vi "Begin.vi"(8 "error in":errorcluster) -> (0 "error out":errorcluster)   [LabVIEW 2019]
doc: "Called before other user functions, this VI is expected to open initial I/O refnums, load in file data, and do all program initialization. Notice that the <B>error out</B> terminal is simply used for data flow. Wiring it to other structures or subVIs ensures that this VI runs first."
uses:
  <vilib>/Rock Robotics/SystemInterfaces/DIO/FPGA_DIOPWMChannel.ctl
  Robot Global Data.vi
  <vilib>/Rock Robotics/WPI/DriverStation/WPI_DriverStationRobotMode2.ctl
  <vilib>/Rock Robotics/WPI/Joystick/WPI_JoystickDeviceEnum.ctl
  <vilib>/Rock Robotics/Network Tables/NT Write String Array.vi
  <vilib>/Rock Robotics/SystemInterfaces/AI/FPGA_AIGyroChannel.ctl
  <vilib>/Rock Robotics/SystemInterfaces/DIO/FPGA_DIOChannel.ctl
  <vilib>/Rock Robotics/WPI/Gyro/WPI_GyroAnalogOpen.vi
  <vilib>/Rock Robotics/WPI/ThirdParty/JAS_Junk/TrajLib/Trajectory_Library.lvlib
panel:
  in  "Tab Control":T1(tab)
  # "Instructions:\nThis should create a path, show the data on the various tabs and optionally write the motor demands and expected results to a file for use on a a robot..\n1) Enter robot data on Robot Data Tab\n2) Define your path definitions.\n3) Define the time increment.  0.020 is chosen since that matches the normal loop time.\n4) Press calculate path.  If a good path was calculated it will be displayed on the Tank Data tab, and the Ready to Execute will indicate execution can begin.\nThe path can be recalculated many times before selecting execute.\n\nTo write to a file.\n5) Select the file name\n6) This example uses \"steps\", sequential numbers for inclusion into a list based autonomous routine.  Including the step number if optional.\n7) This uses command numbers to indicate first, last, and intermediate steps.  This allows some simplification of the execution routine.  It\nalso allows the path to be executed backwards if desired.  The command numbers are changeable.\n8) Press \"Create Command List\".\n\nNotes:\n- PC robot simulataion is disabled in this program.  The code is still there if you want to restore it and try it out.  Use one of the other test programs \nto simulate the path on a PC.\n- The path generation logic doesn't account distribution of speed to the left and right wheels.  As a result the maximum speed can be exceeded.\nIf this happens, but Path Speed > Max light will light and Ready to Execute will not light.  Lower the maximum speed in the Robot Data tab\nand recalulate the path.\n- 2019 playing field size - width: 26 ft 11.25 In = 323.25 in , length: 52 ft 5.25 in = 629.25 in  (I didn't verify this for the 2020 version.)"
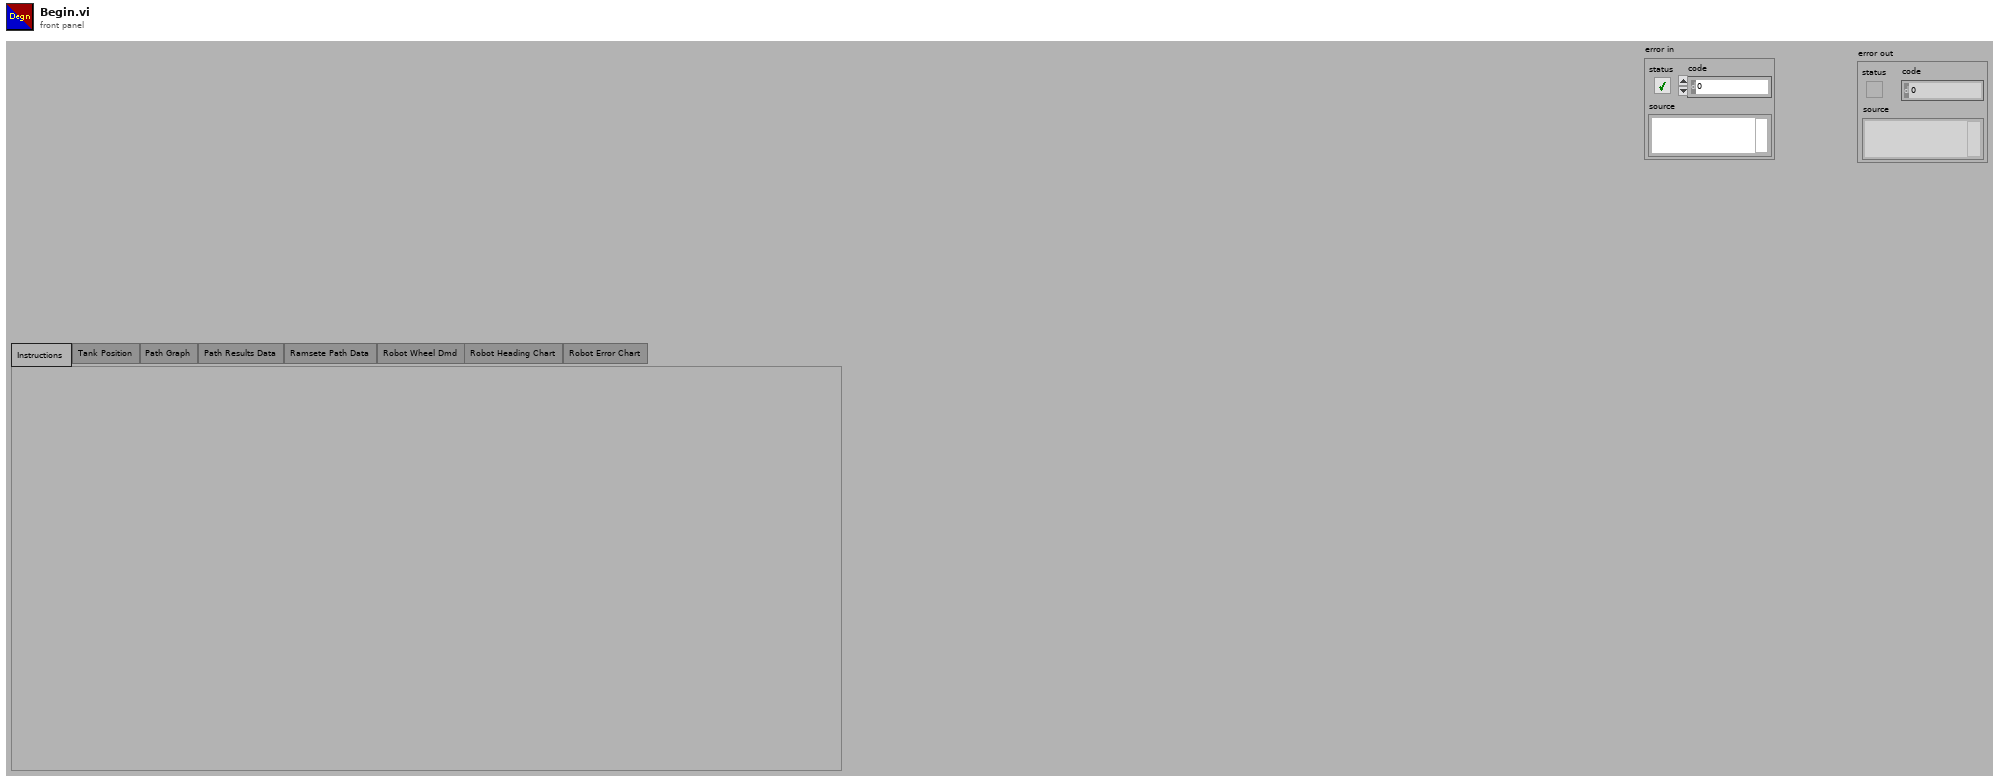
[diagram p1: front panel]
types:
  T1 = enum32{"Instructions", "Tank Position", "Path Graph", "Path Results Data", "Ramsete Path Data", "Robot Wheel Dmd", "Robot Heading Chart", "Robot Error Chart"}
  T2 = typedef "FPGA_DIOChannel.ctl" = enum8{"DIO 0", "DIO 1", "DIO 2", "DIO 3", "DIO 4", "DIO 5", "DIO 6", "DIO 7", "DIO 8", "DIO 9", "DIO MXP 0", "DIO MXP 1", "DIO MXP 2", "DIO MXP 3", "DIO MXP 4", "DIO MXP 5", "DIO MXP 6", "DIO MXP 7", "DIO MXP 8", "DIO MXP 9", "DIO MXP 10", "DIO MXP 11", "DIO MXP 12", "DIO MXP 13", "DIO MXP 14", "DIO MXP 15", "SPI Port CS1", "SPI Port CS2", "SPI Port CS3", "SPI Port MISO", "SPI Port MOSI", "Invalid"}
  T3 = typedef "FPGA_DIOPWMChannel.ctl" = enum8{"PWM 0", "PWM 1", "PWM 2", "PWM 3", "PWM 4", "PWM 5", "PWM 6", "PWM 7", "PWM 8", "PWM 9", "PWM MXP 0", "PWM MXP 1", "PWM MXP 2", "PWM MXP 3", "PWM MXP 4", "PWM MXP 5", "PWM MXP 6", "PWM MXP 7", "PWM MXP 8", "PWM MXP 9", "Invalid"}
  T4 = typedef "FPGA_AIGyroChannel.ctl" = enum8{"AI 0", "AI 1", "Invalid"}
  T5 = typedef "WPI_JoystickDeviceEnum.ctl" = enum16{"USB 0", "USB 1", "USB 2", "USB 3", "USB 4", "USB 5"}
  T6 = typedef "WPI_DriverStationRobotMode2.ctl" = enum16{"Autonomous Disabled", "Autonomous Enabled", "Teleop Disabled", "Teleop Enabled", "Disconnected", "Finish", "Test Disabled", "Test Enabled", "Emergency Stopped"}
  T7 = typedef "Trajectory_Library.lvlib/ROTATION2D.ctl" = cluster{"VALUE":dbl, "COS":dbl, "SIN":dbl}
  T8 = typedef "Trajectory_Library.lvlib/SWERVE_DRIVE_MODULE_POSITION.ctl" = cluster{"Distance":dbl, "Angle":T7, "P":bool}
  T9 = typedef "WPI_JoystickDevRef.ctl" = cluster{"Device":T5}
  T10 = typedef "WPI_GyroDevRef.ctl" = cluster{"DevStatus":errorcluster, "Analog Channel":T11, "Gain (VoltsPerDegree/Second)":dbl, "Gyro Type":enum16{"Analog", "XRS450"}, "Handle":i32, "SPI Bus":T12, "Device Found":bool, "Sample Rate":dbl, "Calibrate On Open":bool, "Offset":dbl}
  T11 = typedef "FPGA_AIChannel.ctl" = enum8{"AI 0", "AI 1", "AI 2", "AI 3", "AI MXP 0", "AI MXP 1", "AI MXP 2", "AI MXP 3", "Invalid"}
  T12 = typedef "spi_bus.ctl" = enum16{"SPI On-Board, CS0", "SPI On-Board, CS1", "SPI On-Board, CS2", "SPI On-Board, CS3", "SPI MXP", "Invalid"}
  T13 = typedef "Trajectory_Library.lvlib/TRANSLATION2D.ctl" = cluster{"X":dbl, "Y":dbl}
  T14 = typedef "Trajectory_Library.lvlib/POSE2D.ctl" = cluster{"TRANSLATION":T13, "ROTATION":T7}
  T15 = typedef "Trajectory_Library.lvlib/SWERVE_DRIVE_ODOMETRY.ctl" = cluster{"POSE":T14, "GyroOffset":T7, "PreviousAngle":T7, "PrevModulePositions":T8[], "NumModules":i32}
  T16 = typedef "Trajectory_Library.lvlib/SWERVE_DRIVE_KINEMATICS.ctl" = cluster{"NumModules":i32, "InverseKinematics":T17, "ForwardKinematics":T17, "Modules":T13[], "PrevCoR":T13, "SavedModuleStates":T18[]}
  T17 = typedef "NI_Matrix.lvlib/RealMatrix.ctl" = dbl[][]
  T18 = typedef "Trajectory_Library.lvlib/SWERVE_DRIVE_MODULE_STATE.ctl" = cluster{"Speed":dbl, "Angle":T7}
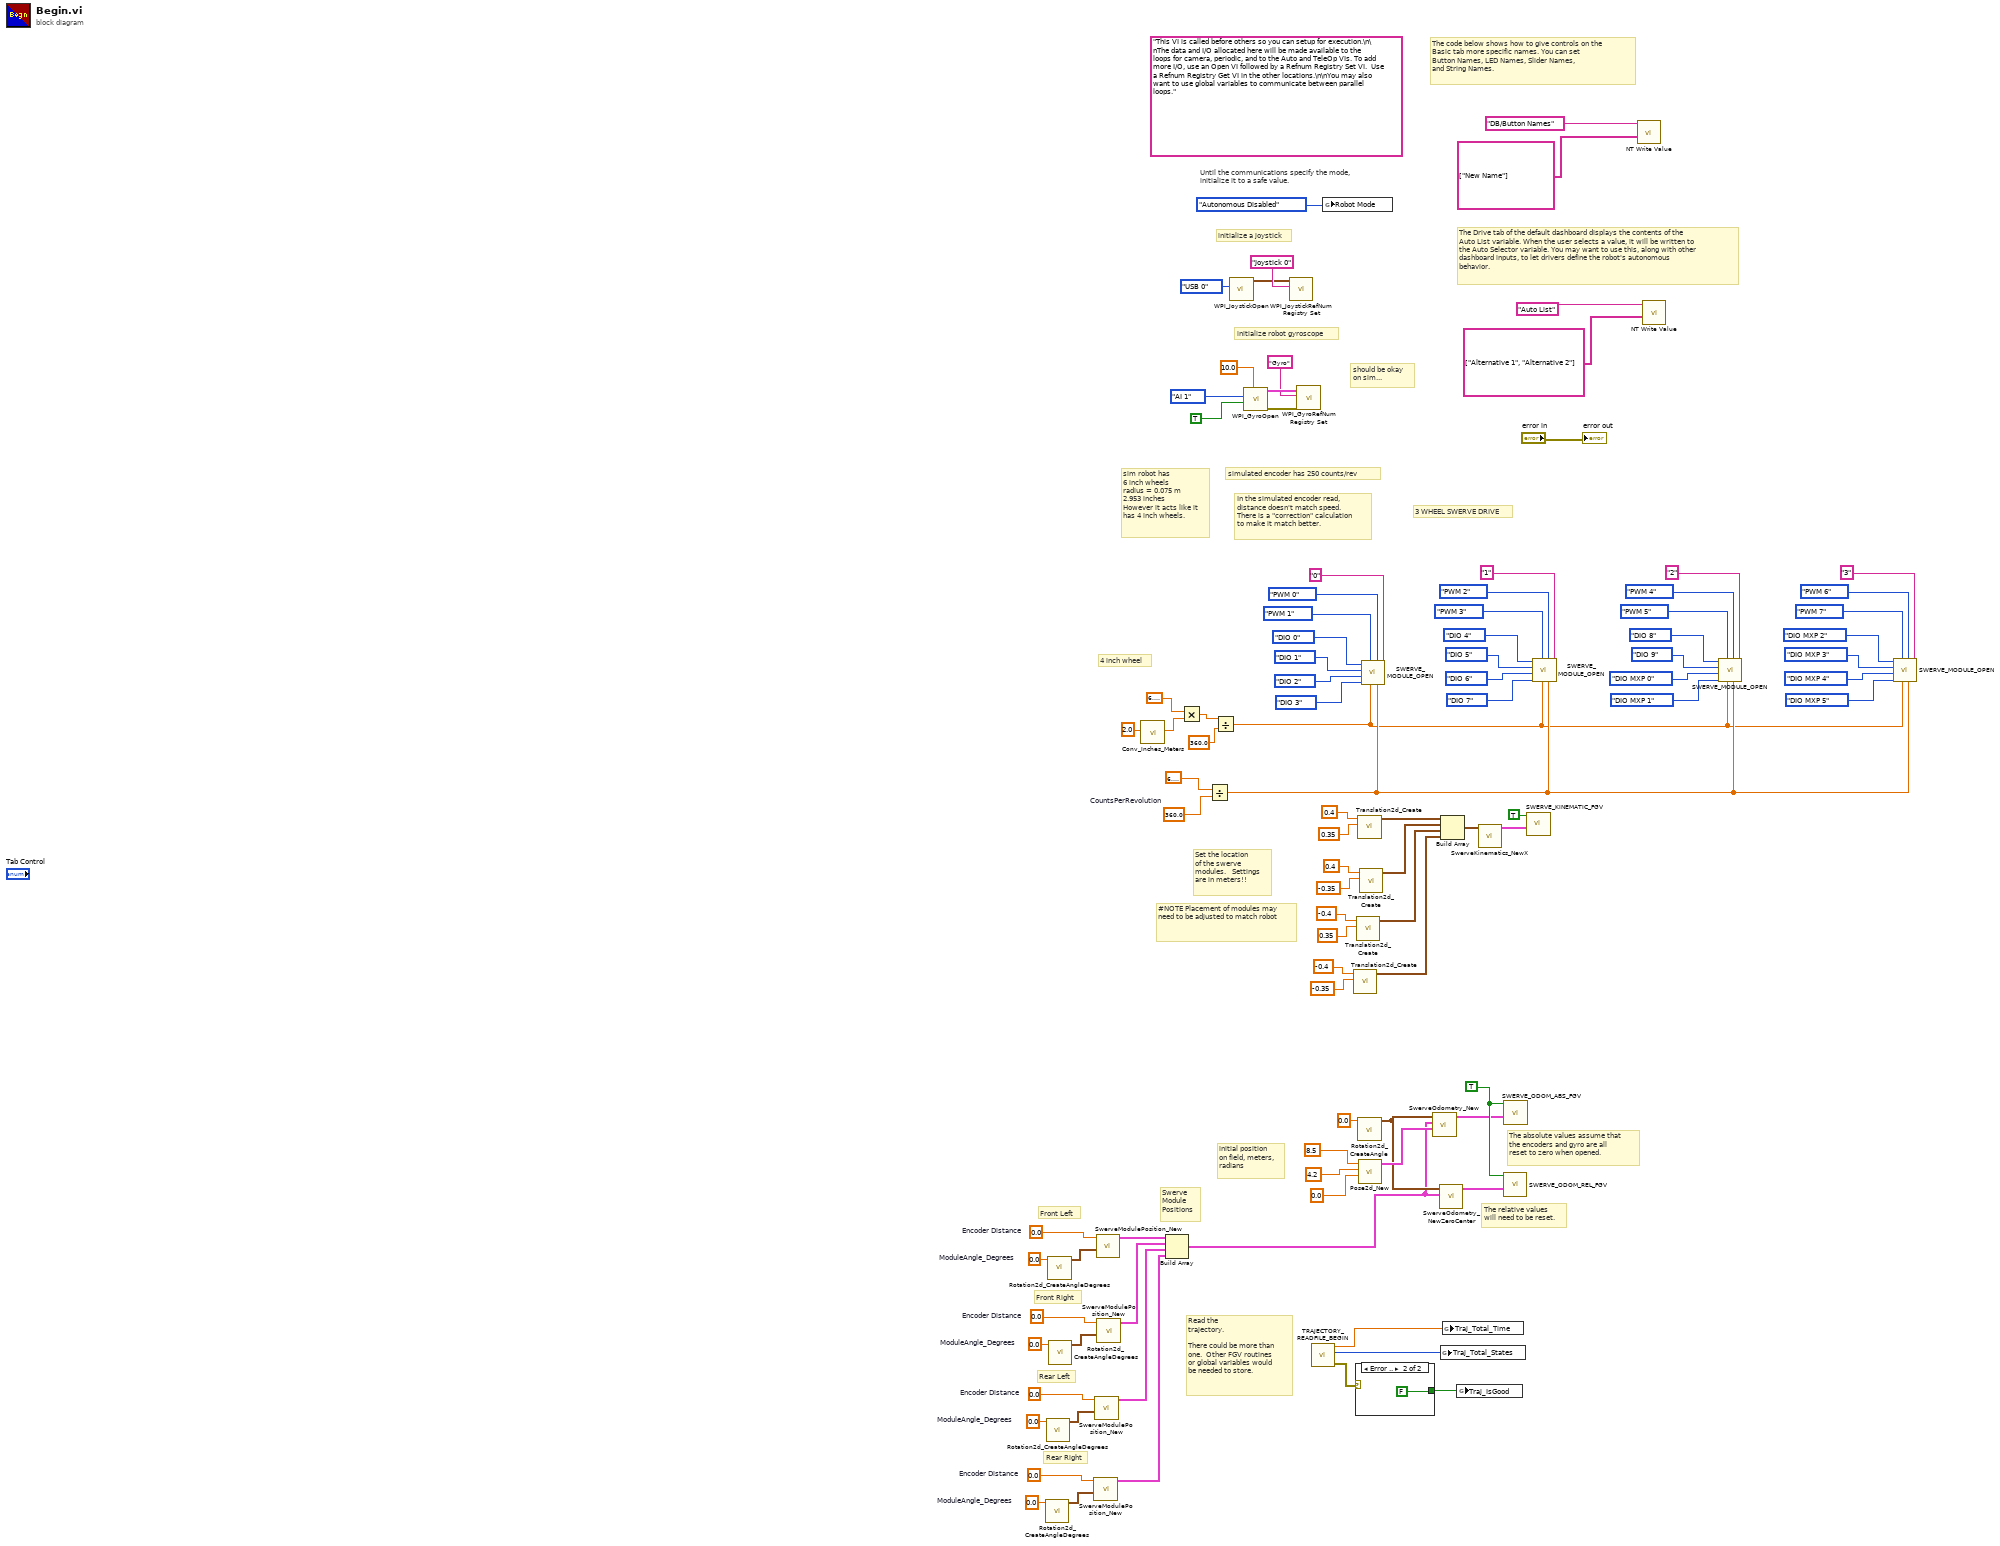
[diagram p0: block diagram]
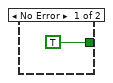
[diagram p2: hidden frame]
diagram:
  w14 = 0.0  # ModuleAngle_Degrees
  w12 = 0.0  # Encoder Distance
  w11 = 0.0  # ModuleAngle_Degrees
  w9 = 0.0  # Encoder Distance
  w8 = 0.0  # ModuleAngle_Degrees
  w6 = 0.0  # Encoder Distance
  w4 = 0.0  # ModuleAngle_Degrees
  w2 = 0.0  # Encoder Distance
  w33 = TRUE ("WRITE")
  w67 = 360.0  # CountsPerRevolution
  (unwired) "This VI is called before others so you can setup for execution.\n\nThe data and I/O allocated here will be made available to the loops for camera, periodic, and to the Auto and TeleOp VIs. To add more I/O, use an Open VI followed by a Refnum Registry Set VI.  Use a Refnum Registry Get VI in the other locations.\n\nYou may also want to use global variables to communicate between parallel loops."
  # "Front Left"
  # "Swerve\nModule\nPositions"
  # "Rear Right"
  # "Rear Left"
  # "Front Right"
  # "#NOTE Placement of modules may need to be adjusted to match robot"
  # "should be okay\non sim..."
  # "The absolute values assume that\nthe encoders and gyro are all\nreset to zero when opened."
  # "The relative values\nwill need to be reset."
  # "initial position\non field, meters,\nradians"
  # "Set the location\nof the swerve \nmodules.   Settings\nare in meters!!"
  # "4 inch wheel"
  # "3 WHEEL SWERVE DRIVE"
  # "initialize robot gyroscope"
  # "Read the\ntrajectory.\n\nThere could be more than\none.  Other FGV routines\nor global variables would\nbe needed to store."
  # "In the simulated encoder read,\ndistance doesn't match speed.\nThere is a \"correction\" calculation\nto make it match better."
  # "simulated encoder has 250 counts/rev"
  # "sim robot has\n6 inch wheels\nradius = 0.075 m\n2.953 inches\nHowever it acts like it\nhas 4 inch wheels."
  # "The Drive tab of the default dashboard displays the contents of the\nAuto List variable. When the user selects a value, it will be written to\nthe Auto Selector variable. You may want to use this, along with other\ndashboard inputs, to let drivers define the robot's autonomous\nbehavior."
  # "The code below shows how to give controls on the\nBasic tab more specific names. You can set\nButton Names, LED Names, Slider Names,\nand String Names."
  # "initialize a joystick"
  # "Until the communications specify the mode,\ninitialize it to a safe value."
  n1 = call <vilib>:"Rotation2d_CreateAngleDegrees.vi"("Angle_Degrees"=w14) -> ("ROTATION"=w13:T7)  [unwired: 10 in]
  n2 = call <vilib>:"Rotation2d_CreateAngleDegrees.vi"("Angle_Degrees"=w11) -> ("ROTATION"=w10:T7)  [unwired: 10 in]
  n3 = call <vilib>:"Rotation2d_CreateAngleDegrees.vi"("Angle_Degrees"=w4) -> ("ROTATION"=w3:T7)  [unwired: 10 in]
  n4 = call <vilib>:"Rotation2d_CreateAngleDegrees.vi"("Angle_Degrees"=w8) -> ("ROTATION"=w7:T7)  [unwired: 10 in]
  n5 = call <vilib>:"SwerveModulePosition_New.vi"("ROTATION"=w13, "Distance"=w12) -> ("SWERVE_DRIVE_MODULE_POSITION"=w17:T8)  [unwired: 9 in]
  n6 = call <vilib>:"SwerveModulePosition_New.vi"("ROTATION"=w10, "Distance"=w9) -> ("SWERVE_DRIVE_MODULE_POSITION"=w16:T8)  [unwired: 9 in]
  n7 = call <vilib>:"SwerveModulePosition_New.vi"("ROTATION"=w3, "Distance"=w2) -> ("SWERVE_DRIVE_MODULE_POSITION"=w5:T8)  [unwired: 9 in]
  n8 = call <vilib>:"SwerveModulePosition_New.vi"("ROTATION"=w7, "Distance"=w6) -> ("SWERVE_DRIVE_MODULE_POSITION"=w15:T8)  [unwired: 9 in]
  n9 = call <vilib>:"Conv_Inches_Meters.vi"("INCH"=2.0) -> ("Meters"=w39:dbl)  [unwired: 10 in]
  n10 = Build Array(w5, w15, w16, w17) -> (w1:T8[])
  n11 = Multiply(x=6.283185307179586, y=w39) -> (x*y=w87:dbl)
  n12 = Divide(x=6.283185307179586, y=w67) -> (x/y=w22:dbl)
  n13 = Divide(x=w87, y=360.0) -> (x/y=w21:dbl)
  n14 = call <vilib>:"WPI_JoystickOpen.vi"("JoystickDevice"=WPI_JoystickDeviceEnum."USB 0") -> ("JoystickDevRef"=w95:T9)  [unwired: 10 in]
  n15 = call-poly <vilib>:"WPI_GyroOpen.vi"("Calibration Time (s)"=10.0, "Calibrate On Open"=TRUE, "Analog Channel"=FPGA_AIGyroChannel."AI 1") -> ("error out"=w84:errorcluster, "GyroDevRef"=w83:T10)  [unwired: 6 in, 1 out]
  n16 = call <vilib>:"WPI_JoystickRefNum Registry Set.vi"("refnum name"="Joystick 0", "JoystickDevRef"=w95) -> ()  [unwired: 8 in, 2 out]
  n17 = call <vilib>:"WPI_GyroRefNum Registry Set.vi"("error in (no error)"=w84, "refnum name"="Gyro", "GyroDevRef"=w83) -> ()  [unwired: 7 in, 2 out]
  n18 = call "TRAJECTORY_READFILE_BEGIN.vi"() -> ("error out"=w81:errorcluster, "Trajectory Items"=w78:i32, "TotalTImeSecs"=w79:dbl)  [unwired: 9 in]
  n19 = global write "Robot Global Data.vi" "Robot Mode"(WPI_DriverStationRobotMode2."Autonomous Disabled" ("Robot Mode")) -> ()
  n20 = call <vilib>:"Translation2d_Create.vi"("Y"=-0.35, "X"=-0.4) -> ("TRANSLATION"=w18:T13)  [unwired: 9 in]
  n21 = case shown="Error .." w81 {
    tunnel: [TRUE FALSE] -> w80
    frame No Error {
    }
    frame Error {
    }
  }
  n22 = call <vilib>:"Translation2d_Create.vi"("Y"=0.35, "X"=-0.4) -> ("TRANSLATION"=w44:T13)  [unwired: 9 in]
  n23 = call <vilib>:"Translation2d_Create.vi"("Y"=0.35, "X"=0.4) -> ("TRANSLATION"=w46:T13)  [unwired: 9 in]
  n24 = call <vilib>:"Rotation2d_CreateAngle.vi"("Angle"=0.0) -> ("ROTATION"=w31:T7)  [unwired: 10 in]
  n25 = call <vilib>:"Pose2d_New.vi"("Heading"=0.0, "Y"=4.2, "X"=8.5) -> ("out POSe"=w34:T14)  [unwired: 8 in]
  n26 = call <vilib>:"Translation2d_Create.vi"("Y"=-0.35, "X"=0.4) -> ("TRANSLATION"=w45:T13)  [unwired: 9 in]
  n27 = call "SWERVE_MODULE_OPEN.vi"("NameSuffix"="0", "RadiansPerCount"=w22, "Drive PWM Channel"=FPGA_DIOPWMChannel."PWM 0", "DistancePerCount"=w21, "Swerve PWM Channel"=FPGA_DIOPWMChannel."PWM 1", "Swerve B Channel"=FPGA_DIOChannel."DIO 3", "Swerver A Channel"=FPGA_DIOChannel."DIO 2", "Drive B Channel"=FPGA_DIOChannel."DIO 1", "Drive A channel"=FPGA_DIOChannel."DIO 0") -> ()  [unwired: 3 in]
  n28 = call <vilib>:"SwerveOdometry_New.vi"("InitialPose"=w34, "Module Positions"=w1, "gyroAngle"=w31) -> ("SWERVE_DRIVE_ODOMETRY"=w32:T15)  [unwired: 8 in]
  n29 = call <vilib>:"SwerveOdometry_NewZeroCenter.vi"("Module Positions"=w1, "gyroAngle"=w31) -> ("SWERVE_DRIVE_ODOMETRY"=w30:T15)  [unwired: 9 in]
  n30 = global write "Robot Global Data.vi" "Traj_Total_States"(w78) -> ()
  n31 = Build Array(w46, w45, w44, w18) -> (w43:T13[])
  n32 = global write "Robot Global Data.vi" "Traj_Total_Time"(w79) -> ()
  n33 = global write "Robot Global Data.vi" "Traj_IsGood"(w80) -> ()
  n34 = call <vilib>:"SwerveKinematics_NewX.vi"("Wheels"=w43) -> ("SWERVE_DRIVE_KINEMATICS"=w41:T16)  [unwired: 10 in]
  n35 = call "SWERVE_ODOM_REL_FGV.vi"("in SWERVE_DRIVE_ODOMETRY"=w30, "WRITE"=w33) -> ()  [unwired: 9 in, 1 out]
  n36 = call "SWERVE_ODOM_ABS_FGV.vi"("in SWERVE_DRIVE_ODOMETRY"=w32, "WRITE"=w33) -> ()  [unwired: 9 in, 1 out]
  n37 = call "SWERVE_KINEMATIC_FGV.vi"("in SWERVE_DRIVE_KINEMATICS"=w41, "WRITE"=TRUE) -> ()  [unwired: 9 in, 1 out]
  n38 = call "SWERVE_MODULE_OPEN.vi"("NameSuffix"="1", "RadiansPerCount"=w22, "Drive PWM Channel"=FPGA_DIOPWMChannel."PWM 2", "DistancePerCount"=w21, "Swerve PWM Channel"=FPGA_DIOPWMChannel."PWM 3", "Swerve B Channel"=FPGA_DIOChannel."DIO 7", "Swerver A Channel"=FPGA_DIOChannel."DIO 6", "Drive B Channel"=FPGA_DIOChannel."DIO 5", "Drive A channel"=FPGA_DIOChannel."DIO 4") -> ()  [unwired: 3 in]
  n39 = call-poly <vilib>:"NT Write Value.vi"("String Array"=string[] ["New Name"], "Name"="DB/Button Names") -> ()  [unwired: 9 in, 1 out]
  n40 = call-poly <vilib>:"NT Write Value.vi"("String Array"=string[] ["Alternative 1", "Alternative 2"], "Name"="Auto List") -> ()  [unwired: 9 in, 1 out]
  n41 = call "SWERVE_MODULE_OPEN.vi"("NameSuffix"="2", "RadiansPerCount"=w22, "Drive PWM Channel"=FPGA_DIOPWMChannel."PWM 4", "DistancePerCount"=w21, "Swerve PWM Channel"=FPGA_DIOPWMChannel."PWM 5", "Swerve B Channel"=FPGA_DIOChannel."DIO MXP 1", "Swerver A Channel"=FPGA_DIOChannel."DIO MXP 0", "Drive B Channel"=FPGA_DIOChannel."DIO 9", "Drive A channel"=FPGA_DIOChannel."DIO 8") -> ()  [unwired: 3 in]
  n42 = call "SWERVE_MODULE_OPEN.vi"("NameSuffix"="3", "RadiansPerCount"=w22, "Drive PWM Channel"=FPGA_DIOPWMChannel."PWM 6", "DistancePerCount"=w21, "Swerve PWM Channel"=FPGA_DIOPWMChannel."PWM 7", "Swerve B Channel"=FPGA_DIOChannel."DIO MXP 5", "Swerver A Channel"=FPGA_DIOChannel."DIO MXP 4", "Drive B Channel"=FPGA_DIOChannel."DIO MXP 3", "Drive A channel"=FPGA_DIOChannel."DIO MXP 2") -> ()  [unwired: 3 in]
  "error out" <- "error in"
